vi "CSC_Tension2Torque.vi"(8 "error in (no error)":errorcluster, 9 "Locked Joints":i32[](array[numeric]), 10 "Cable Tensions":dbl[](array[numeric]), 11 "CSC in":refnum<class "CableSerialChain.lvclass">) -> (0 "error out":errorcluster, 2 "Joint Torque":dbl[](array[numeric]), 3 "CSC out":refnum<class "CableSerialChain.lvclass">)   [LabVIEW 2015, in "CableSerialChain.lvclass"]
uses:
  CableSerialChain.lvclass
  <userlib>/_OpenG.lib/array/array.llb/Delete Elements from 2D Array (DBL)__ogtk.vi
  <vilib>/Analysis/BLAS.llb/dgemv - General Matrix-Vector Product (DBL).vi
  <vilib>/Analysis/NI_AALBLAS.lvlib
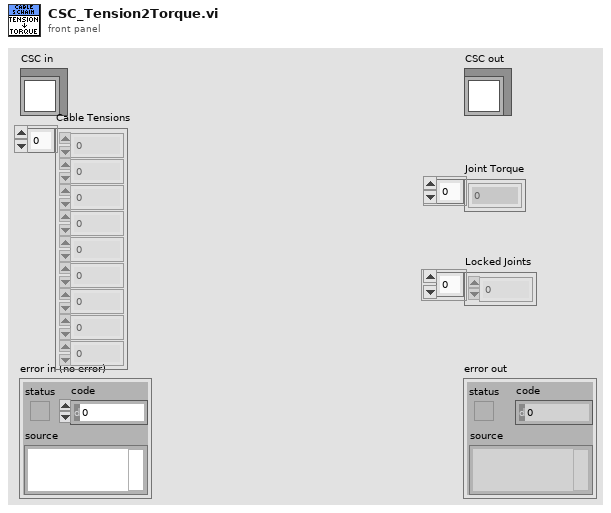
[diagram p1: front panel]
types:
  T1 = typedef "NI_Matrix.lvlib/RealMatrix.ctl" = dbl[][]
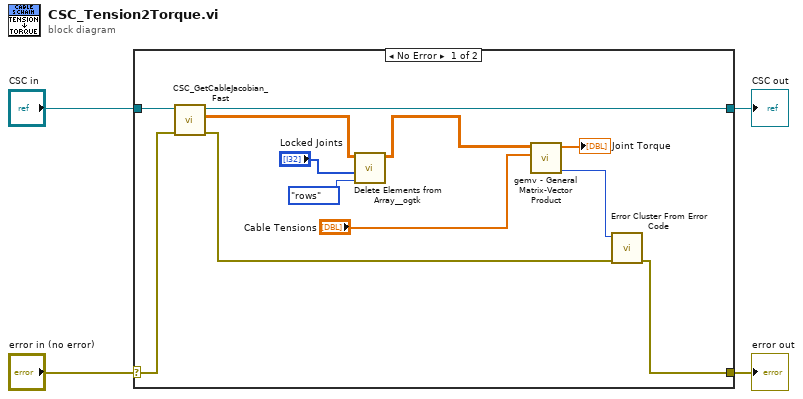
[diagram p0: block diagram]
diagram:
  n1 = case shown="No Error" "error in (no error)" {
    selector: "error in (no error)" -> [w10 w18]
    tunnel: [w14 w18] -> w3
    tunnel: [w11 w17] -> w1
    tunnel: "CSC in" -> [w12 w17]
    frame No Error {
      n2 = call "CSC_GetCableJacobian_Fast.vi"("error in (no error)"=w10, "C-Alex in"=w12) -> ("error out"=w9:errorcluster, "Jacobian for Cables"=w8:T1, "C-Alex out"=w11:refnum<class "CableSerialChain.lvclass">)  [unwired: 7 in]
      n3 = call-poly <userlib>:"Delete Elements from Array__ogtk.vi"("delete (rows or columns)"=enum16{"rows", "columns"}."rows", "indices"="Locked Joints", "array"=w8) -> ("array w/ subset deleted"=w7:dbl[][])  [unwired: 7 in, 1 out]
      n4 = call-poly <vilib>:"gemv - General Matrix-Vector Product.vi"("x"="Cable Tensions", "A"=w7) -> ("error"=w15:i32, "dgemv"=→"Joint Torque":dbl[])  [unwired: 8 in]
      n5 = call <vilib>:"Error Cluster From Error Code.vi"("error in (no error)"=w9, "error code (0)"=w15) -> ("error out"=w14:errorcluster)  [unwired: 7 in]
    }
    frame Error {
    }
  }
  "error out" <- w3
  "CSC out" <- w1
